vi "pR comm loop.vi"(8 "error in (no error)":errorcluster) -> (2 "netw Variable References":T1)   [LabVIEW 2014]
uses:
  Controls/pR Variable References.ctl
  Globals/Global - All Loop Stop.vi
  Globals/Global - pR netw comm.vi
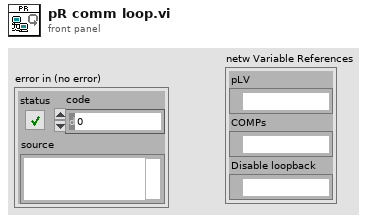
[diagram p1: front panel]
types:
  T1 = typedef "pR Variable References.ctl" = cluster{"pLV":refnum<k21>, "COMPs":refnum<k21>, "Disable loopback":refnum<k21>}
  T2 = enum16{"reconnect wait", "connected", "disconnected"}
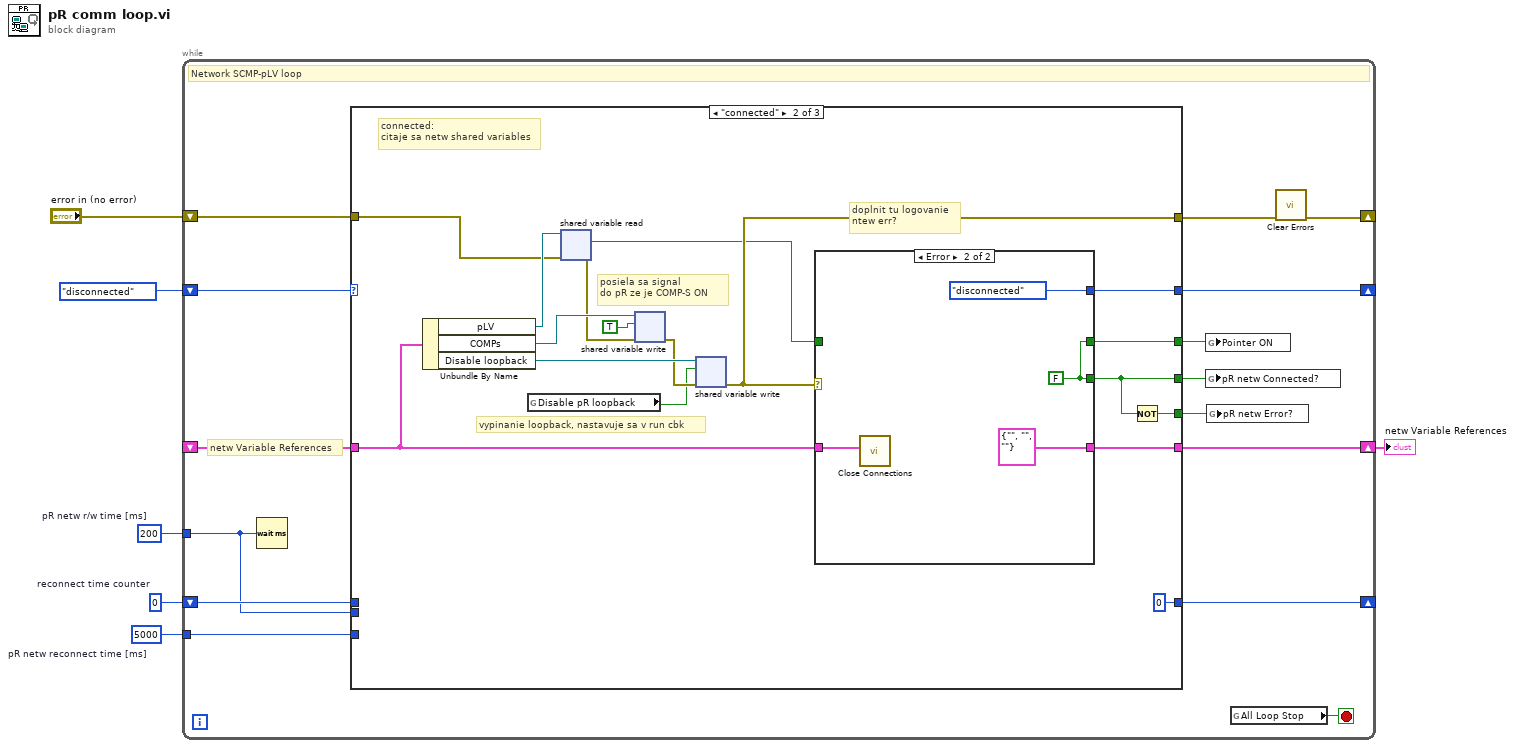
[diagram p0: block diagram]
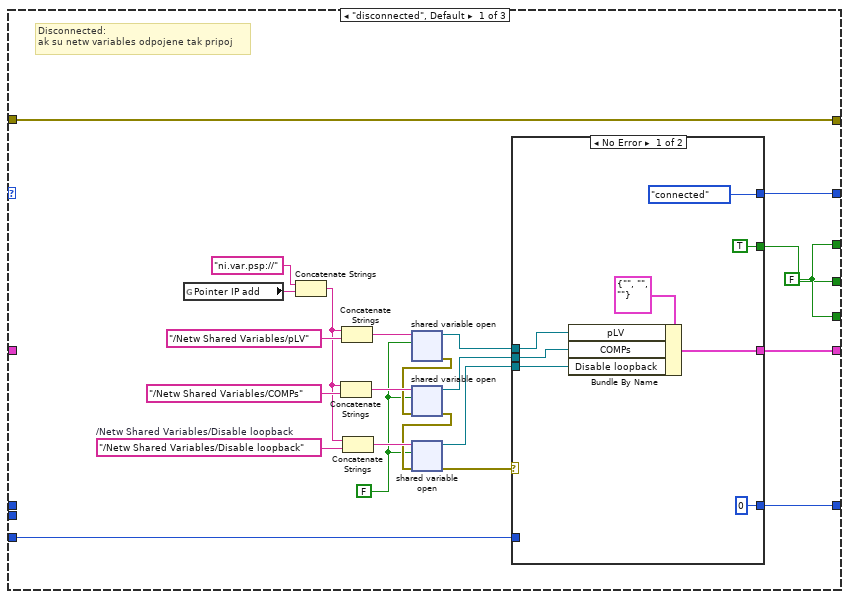
[diagram p2: hidden frame]
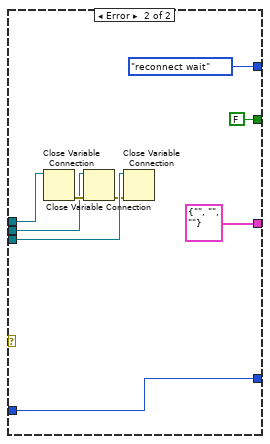
[diagram p3: hidden frame]
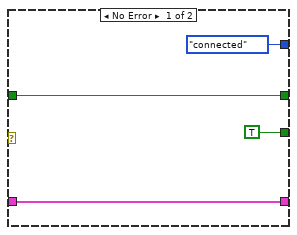
[diagram p4: hidden frame]
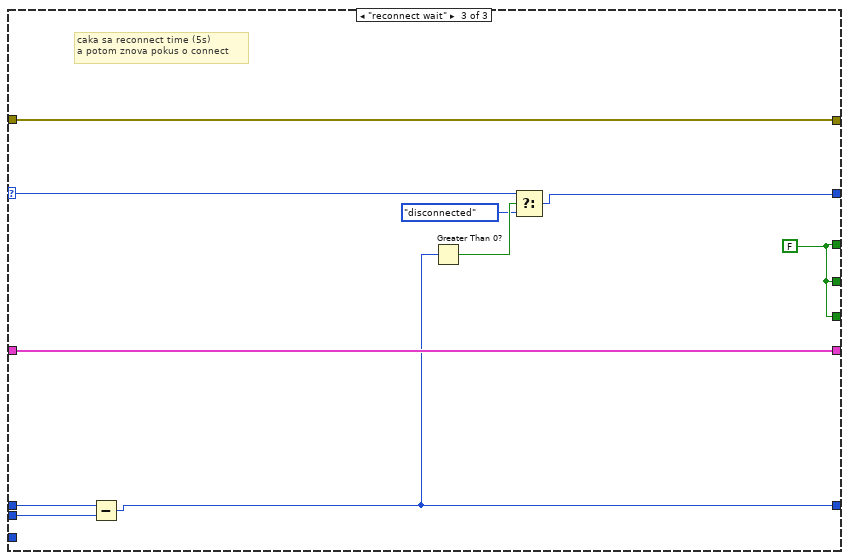
[diagram p5: hidden frame]
diagram:
  w1 = u32 0  # reconnect time counter
  w4 = u32 5000  # pR netw reconnect time [ms]
  w5 = u32 200  # pR netw r/w time [ms]
  n1 = while {
    tunnel: w5 -> [w7]
    shift-right: [w18] -> _
    shift-left: "error in (no error)" -> [w19]
    shift-right: [w17] -> w3
    shift-left: _ -> [w16]
    tunnel: w4 -> [w14]
    shift-right: [w10] -> _
    shift-left: T2."disconnected" -> [w11]
    shift-right: [w9] -> _
    shift-left: w1 -> [w8]
    stop <- w21 stop-if-true
    # "netw Variable References"
    # "Network SCMP-pLV loop"
    n2 = Wait (ms)(milliseconds to wait=w7) -> ()  [unwired: 1 out]
    n3 = case shown="\"connected\"" w11 {
      selector: w11 -> [_ _ w89]
      tunnel: [w44 w70 w96] -> w20
      tunnel: w19 -> [w44 w71 w96]
      tunnel: [w27 w69 w92] -> w17
      tunnel: w16 -> [_ w68 w92]
      tunnel: [w24 w65 w93] -> w15
      tunnel: w14 -> [w23 _ _]
      tunnel: [w26 w63 w93] -> w13
      tunnel: [w26 w67 w93] -> w12
      tunnel: [w25 w66 w88] -> w10
      tunnel: [w22 u32 0 ("pR netw reconnect time [ms]") w91] -> w9
      tunnel: w8 -> [_ _ w95]
      tunnel: w7 -> [_ _ w94]
      frame "disconnected", Default {
        w30 = FALSE (".not. x?")
        w37 = "/Netw Shared Variables/Disable loopback"  # /Netw Shared Variables/Disable loopback
        w26 = FALSE ("Pointer ON")
        # "Disconnected:\nak su netw variables odpojene tak pripoj"
        n4 = global read "Global - pR netw comm.vi" "Pointer IP add"() -> (w28:string)
        n5 = Concatenate Strings("ni.var.psp://", w28) -> (w32:string)
        n6 = Concatenate Strings(w32, "/Netw Shared Variables/COMPs") -> (w39:string)
        n7 = Concatenate Strings(w32, "/Netw Shared Variables/pLV") -> (w42:string)
        n8 = Concatenate Strings(w32, w37) -> (w38:string)
        n9 = shared-variable-open(w42, w30) -> (w35:refnum<k21>, w36:errorcluster)  [unwired: 2 in]
        n10 = shared-variable-open(w39, w36, w30) -> (w34:refnum<k21>, w31:errorcluster)  [unwired: 1 in]
        n11 = shared-variable-open(w38, w31, w30) -> (w33:refnum<k21>, w29:errorcluster)  [unwired: 1 in]
        n12 = case shown="No Error" w29 {
          tunnel: w35 -> [w52 w60]
          tunnel: w34 -> [w50 w58]
          tunnel: w33 -> [w49 w59]
          tunnel: [w48 T1 {"pLV"="", "COMPs"="", "Disable loopback"=""} ("Variable References")] -> w27
          tunnel: [T2."connected" T2."reconnect wait"] -> w25
          tunnel: [TRUE (".not. x?") FALSE (".not. x?")] -> w24
          tunnel: w23 -> [_ w53]
          tunnel: [u32 0 ("pR netw reconnect time [ms]") w53] -> w22
          frame No Error {
            # "Connection successfully established."
            n13 = Bundle By Name(cluster=T1 {"pLV"="", "COMPs"="", "Disable loopback"=""} ("Variable References"), "pLV"=w52, "COMPs"=w50, "Disable loopback"=w49) -> (w48:T1)
          }
          frame Error {
            # "An error occurred while connecting. Close all the attempted connection references."
            n14 = Close Variable Connection(11:w60) -> (0:w61:errorcluster)  [unwired: 1 in]
            n15 = Close Variable Connection(8:w61, 11:w58) -> (0:w57:errorcluster)
            n16 = Close Variable Connection(8:w57, 11:w59) -> ()  [unwired: 1 out]
          }
        }
      }
      frame "connected" {
        # "connected:\ncitaje sa netw shared variables"
        # "vypinanie loopback, nastavuje sa v run cbk"
        # "posiela sa signal\ndo pR ze je COMP-S ON"
        # "doplnit tu logovanie\nntew err?"
        n17 = Unbundle By Name(w68) -> ("pLV"=w78:refnum<k21>, "COMPs"=w77:refnum<k21>, "Disable loopback"=w75:refnum<k21>)
        n18 = global read "Global - pR netw comm.vi" "Disable pR loopback"() -> (w73:bool)
        n19 = shared-variable-read(w78, w71) -> (w72:errorcluster, w62:bool)  [unwired: 2 out]
        n20 = shared-variable-write(w77, w72, TRUE ("data in")) -> (w74:errorcluster)  [unwired: 1 out]
        n21 = shared-variable-write(w75, w74, w73) -> (w70:errorcluster)  [unwired: 1 out]
        n22 = case shown="Error" w70 {
          tunnel: [w82 T1 {"pLV"="", "COMPs"="", "Disable loopback"=""} ("Variable References")] -> w69
          tunnel: w68 -> [w82 w85]
          tunnel: [TRUE ("Pointer ON") w83] -> w65
          tunnel: [T2."connected" T2."disconnected"] -> w66
          tunnel: [w79 w83] -> w63
          tunnel: w62 -> [w79 _]
          frame No Error {
          }
          frame Error {
            w83 = FALSE ("Pointer ON")
            n23 = call "Close Connections.vi"("netw Variable References"=w85) -> ()  [unwired: 11 in]
          }
        }
        n24 = Not(x=w65) -> (.not. x?=w67:bool)
      }
      frame "reconnect wait" {
        w93 = FALSE ("Pointer ON")
        # "caka sa reconnect time (5s)\na potom znova pokus o connect"
        n25 = Subtract(x=w95, y=w94) -> (x-y=w91:u32)
        n26 = Greater Than 0?(x=w91) -> (x > 0?=w90:bool)
        n27 = Select(t=w89, s=w90, f=T2."disconnected") -> (s? t:f=w88:T2)
      }
    }
    n28 = global write "Global - pR netw comm.vi" "Pointer ON"(w13) -> ()
    n29 = global write "Global - pR netw comm.vi" "pR netw Connected?"(w15) -> ()
    n30 = global write "Global - pR netw comm.vi" "pR netw Error?"(w12) -> ()
    n31 = global read "Global - All Loop Stop.vi" "All Loop Stop"() -> (w21:bool)
    n32 = call <vilib>:"Clear Errors.vi"("error in (no error)"=w20) -> ("error out"=w18:errorcluster)  [unwired: 5 in, 1 out]
  }
  "netw Variable References" <- w3
